vi "ServerMYiTOPS_DEMO.vi"() -> ()   [LabVIEW 2017]
doc: "Demonstrates how to set up a basic TCP connection, send data to the specified port once a connection has been established, and terminate the connection once the data has been sent. This VI is designed to stop if the TCP connection is terminated. The data sent in this example is an array of random numbers."
panel:
  out "remote address":string
  in  "Virtual Switch":bool
  out "Virtual LED":bool
  in  "Client Closed":string="The client VI closed the connection."
  out "Waveform Graph":dbl[](graph)
  in  "Stop":bool
  # "This server is a modification of LabVIEW sample project \"Simple TCP.lvproj\"."
  # "Overview: Demonstrates the use of the TCP functions to initialize a TCP server that can send data to a client VI.\nInstructions:\n1. Run the VI.\n2. Open Simple TCP - Client.vi and follow the instructions on its front panel. Note that if you wait longer than 30 seconds to do this after running this VI, it will time out.\n3. Click Stop to stop the VI. Note that if you stop the client VI, this VI will stop automatically."
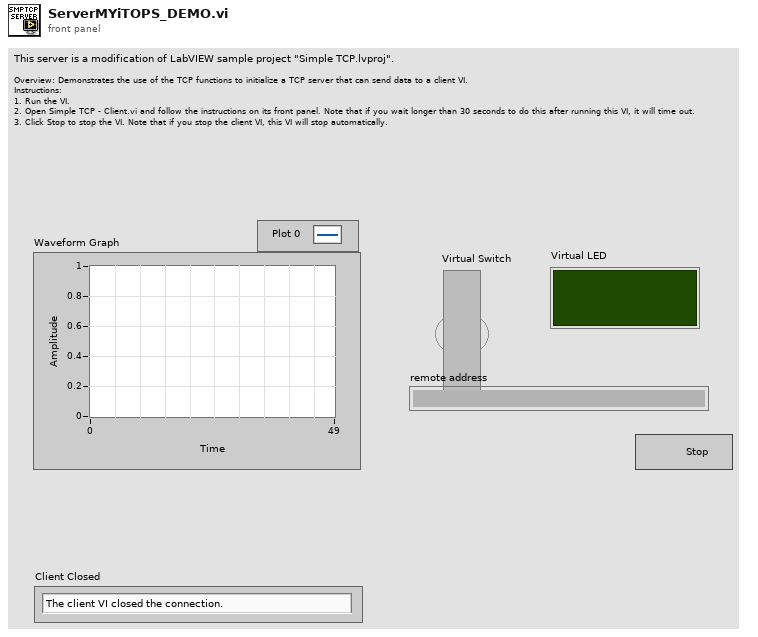
[diagram p1: front panel]
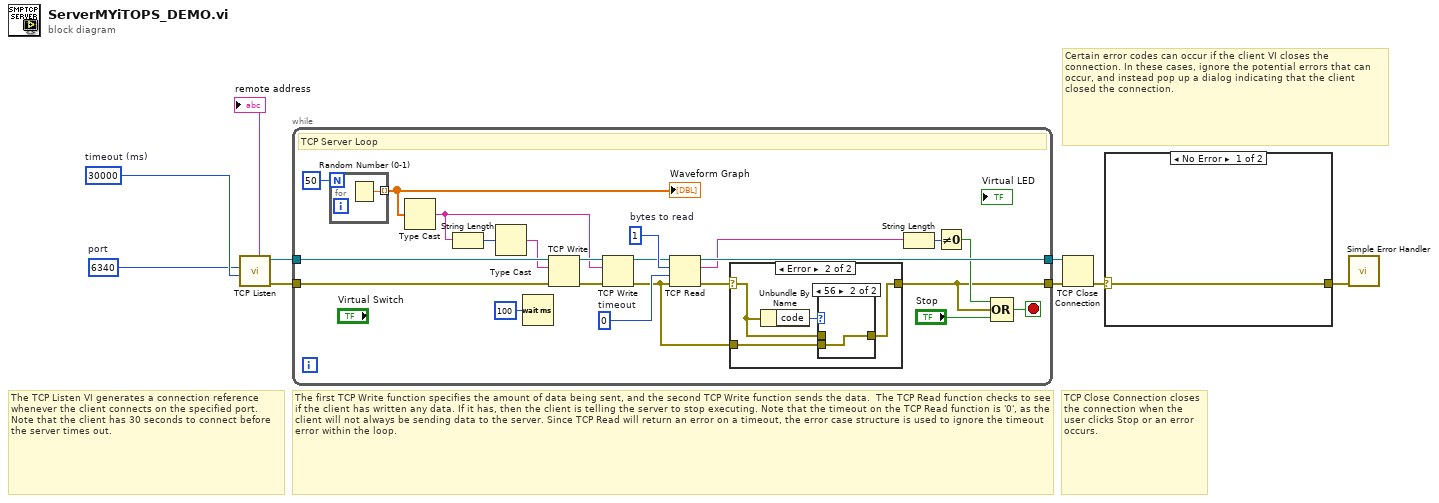
[diagram p0: block diagram]
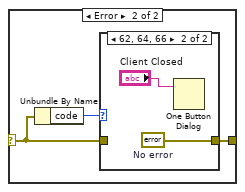
[diagram p2: hidden frame]
diagram:
  w2 = u16 6340  # port
  w3 = 30000  # timeout (ms)
  # "TCP Close Connection closes the connection when the user clicks Stop or an error occurs."
  # "The TCP Listen VI generates a connection reference whenever the client connects on the specified port. Note that the client has 30 seconds to connect before the server times out."
  # "Certain error codes can occur if the client VI closes the connection. In these cases, ignore the potential errors that can occur, and instead pop up a dialog indicating that the client closed the connection."
  # "The first TCP Write function specifies the amount of data being sent, and the second TCP Write function sends the data.  The TCP Read function checks to see if the client has written any data. If it has, then the client is telling the server to stop executing. Note that the timeout on the TCP Read function is '0', as the client will not always be sending data to the server. Since TCP Read will return an error on a timeout, the error case structure is used to ignore the timeout error within the loop."
  n1 = call <vilib>:"TCP Listen.vi"("timeout ms (wait forever: -1)"=w3, "port"=w2) -> ("error out"=w4:errorcluster, "remote address"=→"remote address":string, "connection ID"=w5:refnum<k5>)  [unwired: 5 in, 2 out]
  n2 = while {
    tunnel: [w11] -> w8
    tunnel: [w17] -> w9
    tunnel: w5 -> [w31]
    tunnel: w4 -> [w22]
    stop <- w24 stop-if-true
    w16 = 0  # timeout
    w19 = 1  # bytes to read
    # "TCP Server Loop"
    n3 = for {
      N: 50 ("# of Points") -> [_]
      tunnel: [w39] -> w20 mode=indexing
      n4 = Random Number (0-1)() -> (number: 0 to 1=w39:dbl)
    }
    "Waveform Graph" <- w20
    n5 = Type Cast(x=w20) -> (*(type *) &x=w26:string)  [unwired: 1 out]
    n6 = String Length(string=w26) -> (length=w28:i32)
    n7 = Type Cast(x=w28) -> (*(type *) &x=w27:string)  [unwired: 1 out]
    n8 = Wait (ms)(milliseconds to wait=u32 100) -> ()  [unwired: 1 out]
    n9 = TCP Write(connection ID=w31, data in=w27, error in (no error)=w22) -> (connection ID out=w30:refnum<k5>, error out=w29:errorcluster)  [unwired: 2 out]
    n10 = TCP Write(connection ID=w30, data in=w26, error in (no error)=w29) -> (connection ID out=w18:refnum<k5>, error out=w10:errorcluster)  [unwired: 2 out]
    n11 = TCP Read(connection ID=w18, bytes to read=w19, error in (no error)=w10, 9:w16) -> (connection ID out=w17:refnum<k5>, data out=w14:string, error out=w12:errorcluster)  [unwired: 1 out]
    n12 = case shown="Error" w12 {
      selector: w12 -> [w32 w35]
      tunnel: [w32 w33] -> w11
      tunnel: w10 -> [_ w34]
      frame No Error {
      }
      frame Error {
        n13 = Unbundle By Name(w35) -> ("code"=w36:i32)
        n14 = case shown="56" w36 {
          tunnel: w35 -> [w37 _]
          tunnel: w34 -> [_ w38]
          tunnel: [w37 w38] -> w33
          frame Default {
          }
          frame 56 {
          }
        }
      }
    }
    n15 = String Length(string=w14) -> (length=w15:i32)
    n16 = Not Equal To 0?(x=w15) -> (x != 0?=w13:bool)
    n17 = Compound Arithmetic op=OR(w13, w11, "Stop") -> (w24:bool)
  }
  n18 = TCP Close Connection(connection ID=w9, error in (no error)=w8) -> (error out=w7:errorcluster)  [unwired: 2 out]
  n19 = case shown="No Error" w7 {
    selector: w7 -> [w40 w42]
    tunnel: [w40 w41] -> w6
    frame No Error {
    }
    frame Error {
      n20 = Unbundle By Name(w42) -> ("code"=w43:i32)
      n21 = case shown="62, 64, 66" w43 {
        tunnel: w42 -> [w44 _]
        tunnel: [w44 w46] -> w41
        frame Default {
        }
        frame 62, 64, 66 {
          w46 = errorcluster {"status"=FALSE, "code"=0, "source"=""}  # No error
          n22 = One Button Dialog(message="Client Closed") -> ()  [unwired: 1 in, 1 out]
        }
      }
    }
  }
  n23 = call <vilib>:"Simple Error Handler.vi"("error in (no error)"=w6) -> ()  [unwired: 1 in, 8 out]
